vi "ControlSubMM.vi"(0 "ControlPara":dbl[][](array[numeric]), 1 "AxisForceSample":dbl[](array[numeric]), 2 "ChannelSetArray":T1[](array[typedef]) {"Enable" items=["不使能", "使能"]; "Wave" items=["0指令", "正弦波", "方波", "三角波", "常值", "波形数据", "白噪声", "正弦扫频", "梯度加载", "VMIC"]; "ChannelType" items=["标准波形跟踪"=1, "扫频测试"=2, "消除多余力"=3, "梯度加载"=4, "载荷谱跟踪"=5, "模拟输入跟踪"=9]; "ChannelStatus" items=["通道关", "位置通道", "加载通道"]}, 3 "syn-error":dbl[](array[numeric]), 5 "Angel":bool[](array[boolean]), 7 "TorqueSample":dbl[](array[numeric]), 9 "Command":dbl[](array[numeric]), 12 "dt":dbl, 13 "Torque":bool[](array[boolean]), 14 "AngleSample":dbl[](array[numeric])) -> (4 "数组":dbl[](array[numeric]))   [LabVIEW 2020]
uses:
  ChannelCommand.ctl
  Control 1.ctl
  WaveType.ctl
  MoterEnable.ctl
  <vilib>/addons/control/pid/pid.llb/PID (DBL Array).vi
  <vilib>/addons/control/pid/NI_PID_pid.lvlib
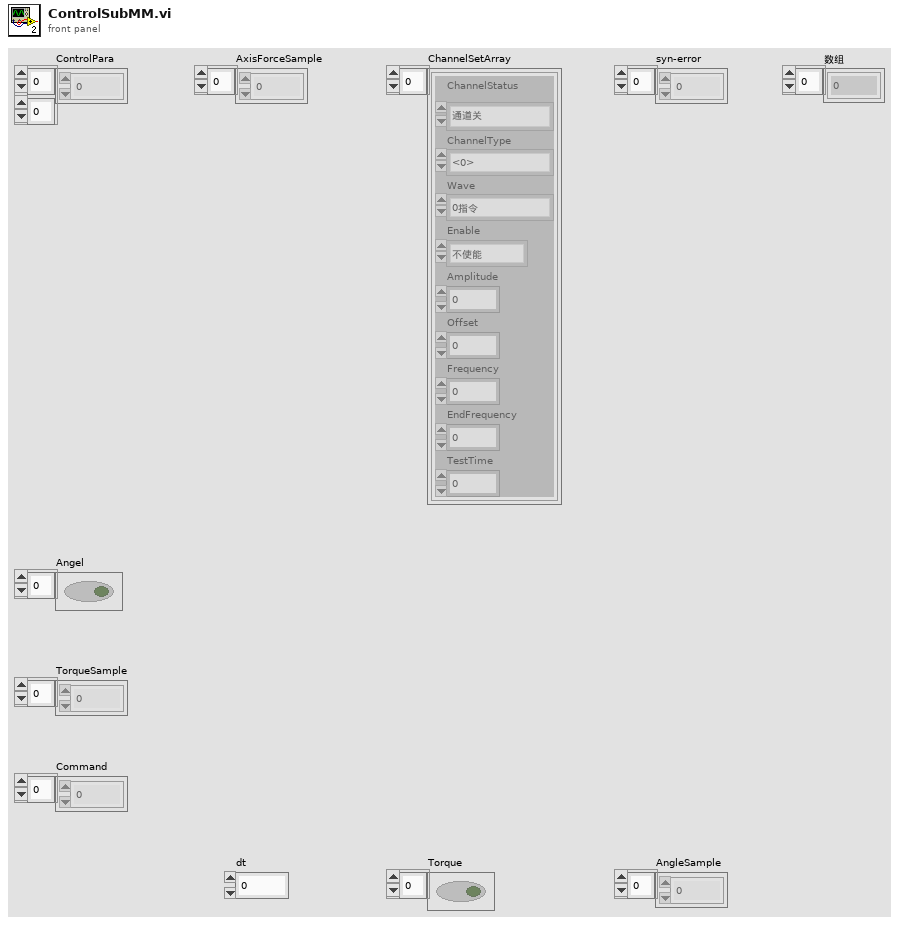
[diagram p1: front panel]
types:
  T1 = typedef "ChannelCommand.ctl" = cluster{"ChannelStatus":T2, "ChannelType":i32, "Wave":T3, "Enable":T4, "Amplitude":dbl, "Offset":dbl, "Frequency":dbl, "EndFrequency":dbl, "TestTime":dbl}
  T2 = typedef "Control 1.ctl" = i32
  T3 = typedef "WaveType.ctl" = i32
  T4 = typedef "MoterEnable.ctl" = u16
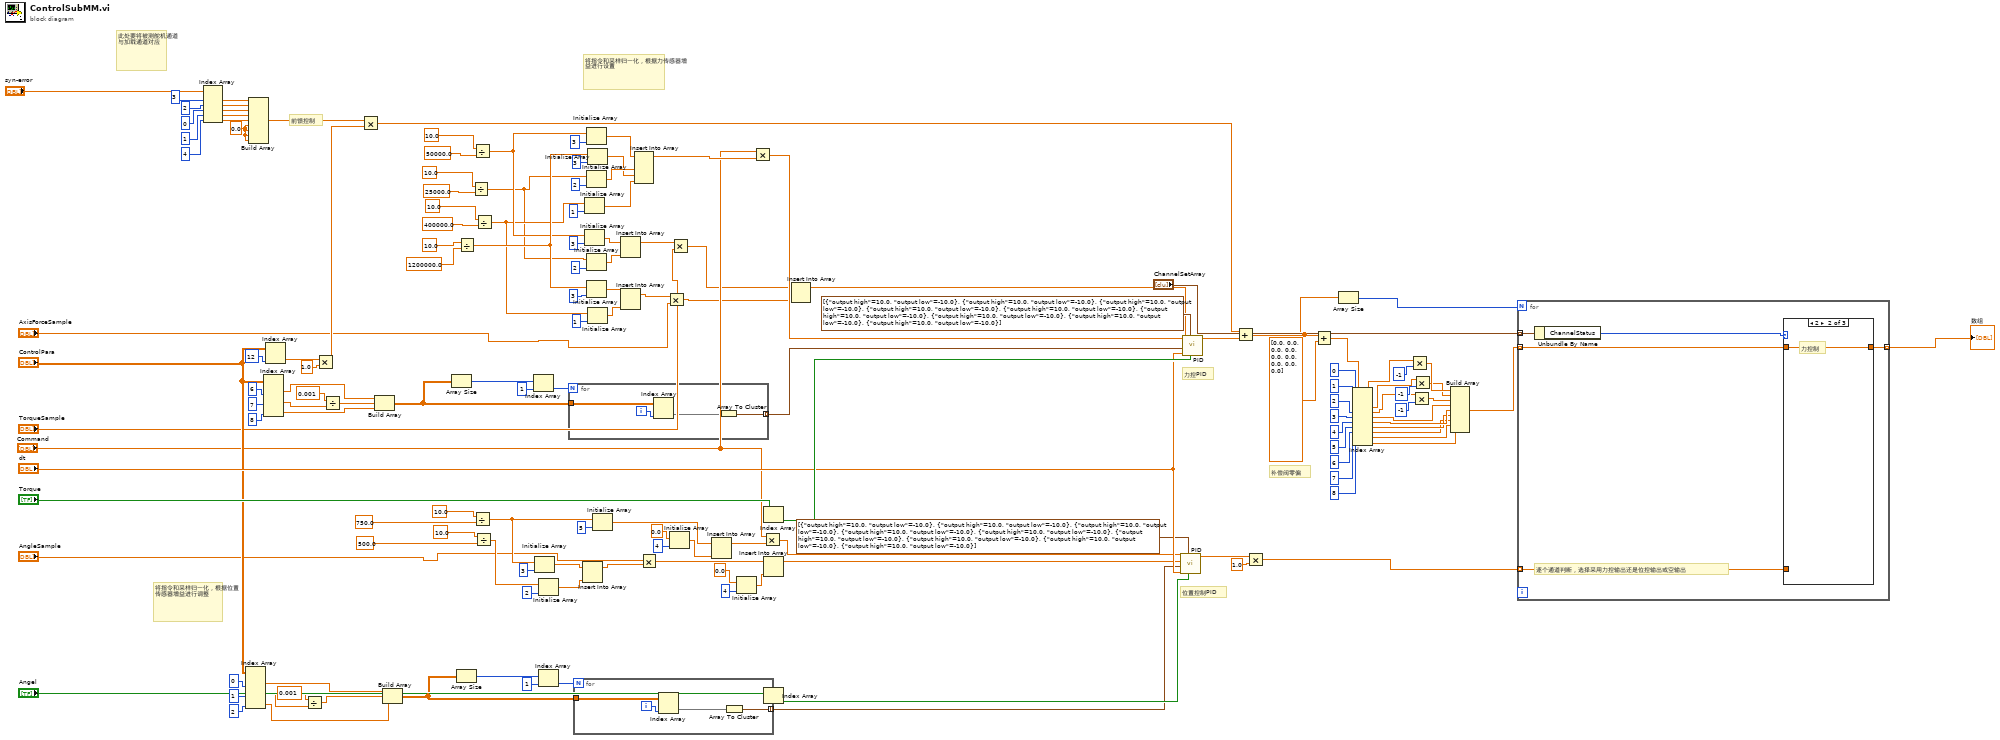
[diagram p0: block diagram]
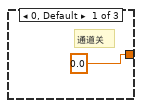
[diagram p2: hidden frame]
diagram:
  w94 = 0.0
  # "补偿阀零偏"
  # "此处要将被测舵机通道与加载通道对应"
  # "将指令和采样归一化，根据力传感器增益进行设置"
  # "将指令和采样归一化，根据位置传感器增益进行调整"
  # "位置控制PID"
  # "力控PID"
  # "前馈控制"
  n1 = Index Array(array="syn-error", index #1=3 ("索引"), index #2=2 ("索引"), index #3=0 ("索引"), index #4=1 ("索引"), index #5=4 ("索引")) -> (element #1=w89:dbl, element #2=w90:dbl, element #3=w91:dbl, element #4=w92:dbl, element #5=w93:dbl)
  n2 = Index Array(array="ControlPara", index (col) #1=0 ("禁用的索引 (列)"), index (col) #2=1 ("索引 (列)"), index (col) #3=2 ("索引 (列)")) -> (element #1=w108:dbl[], element #2=w123:dbl[], element #3=w109:dbl[])  [unwired: 3 in]
  n3 = Build Array(w89, w90, w91, w92, w93, w94, w94, w94, w94) -> (w97:dbl[])
  n4 = Index Array(array="ControlPara", index (col) #1=6 ("禁用的索引 (列)"), index (col) #2=7 ("索引 (列)"), index (col) #3=8 ("索引 (列)")) -> (element #1=w73:dbl[], element #2=w120:dbl[], element #3=w74:dbl[])  [unwired: 3 in]
  n5 = Index Array(array="ControlPara", index (col)=12 ("禁用的索引 (列)")) -> (element=w82:dbl[])  [unwired: 1 in]
  n6 = Divide(x=0.001, y=w123) -> (x/y=w124:dbl[])
  n7 = Multiply(x=w82, y=1.0) -> (x*y=w96:dbl[])
  n8 = Divide(x=0.001, y=w120) -> (x/y=w121:dbl[])
  n9 = Multiply(x=w97, y=w96) -> (x*y=w140:dbl[])
  n10 = Build Array(w73, w121, w74) -> (w78:dbl[][])
  n11 = Build Array(w108, w124, w109) -> (w113:dbl[][])
  n12 = Array Size(array=w78) -> (size(s)=w75:i32[])
  n13 = Array Size(array=w113) -> (size(s)=w110:i32[])
  n14 = Divide(x=10.0 ("元素"), y=1200000.0) -> (x/y=w144:dbl)
  n15 = Divide(x=10.0 ("元素"), y=25000.0) -> (x/y=w44:dbl)
  n16 = Divide(x=10.0 ("元素"), y=50000.0) -> (x/y=w125:dbl)
  n17 = Divide(x=10.0 ("元素"), y=750.0) -> (x/y=w149:dbl)
  n18 = Divide(x=10.0 ("元素"), y=500.0) -> (x/y=w58:dbl)
  n19 = Divide(x=10.0 ("元素"), y=400000.0) -> (x/y=w45:dbl)
  n20 = Index Array(array=w75, index=1 ("索引")) -> (element=w77:i32)
  n21 = Initialize Array(w149, 3 ("维数大小")) -> (w57:dbl[])
  n22 = Initialize Array(w58, 2 ("维数大小")) -> (w56:dbl[])
  n23 = Index Array(array=w110, index=1 ("索引")) -> (element=w112:i32)
  n24 = for {
    N: w77 -> [_]
    tunnel: w78 -> [w153]
    tunnel: [w150] -> w79 mode=indexing
    i -> [w151]
    n25 = Index Array(array=w153, index (col)=w151) -> (element=w152:dbl[])  [unwired: 1 in]
    n26 = Array To Cluster(array=w152) -> (cluster=w150:cluster{"[0]":dbl, "[1]":dbl, "[2]":dbl})
  }
  n27 = for {
    N: w112 -> [_]
    tunnel: w113 -> [w157]
    tunnel: [w154] -> w114 mode=indexing
    i -> [w155]
    n28 = Index Array(array=w157, index (col)=w155) -> (element=w156:dbl[])  [unwired: 1 in]
    n29 = Array To Cluster(array=w156) -> (cluster=w154:cluster{"[0]":dbl, "[1]":dbl, "[2]":dbl})
  }
  n30 = Insert Into Array(array=w57, new element=w56) -> (w55:dbl[])  [unwired: 1 in]
  n31 = Initialize Array(w45, 1 ("维数大小")) -> (w41:dbl[])
  n32 = Initialize Array(w125, 3 ("维数大小")) -> (w38:dbl[])
  n33 = Initialize Array(w125, 3 ("维数大小")) -> (w42:dbl[])
  n34 = Initialize Array(w144, 3 ("维数大小")) -> (w36:dbl[])
  n35 = Initialize Array(w44, 2 ("维数大小")) -> (w40:dbl[])
  n36 = Initialize Array(w44, 2 ("维数大小")) -> (w37:dbl[])
  n37 = Initialize Array(w144, 3 ("维数大小")) -> (w39:dbl[])
  n38 = Initialize Array(w45, 1 ("维数大小")) -> (w35:dbl[])
  n39 = Initialize Array(w149, 5 ("维数大小")) -> (w100:dbl[])
  n40 = Insert Into Array(array=w38, new element=w37) -> (w33:dbl[])  [unwired: 1 in]
  n41 = Insert Into Array(array=w36, new element=w35) -> (w30:dbl[])  [unwired: 1 in]
  n42 = Insert Into Array(array=w42, new element #1=w40, new element #2=w39, new element #3=w41) -> (w63:dbl[])  [unwired: 1 in]
  n43 = Multiply(x="AngleSample", y=w55) -> (x*y=w132:dbl[])
  n44 = Multiply(x=w30, y="AxisForceSample") -> (x*y=w28:dbl[])
  n45 = Initialize Array(0.0 ("元素"), 4 ("维数大小")) -> (w127:dbl[])
  n46 = Multiply(x=w33, y="TorqueSample") -> (x*y=w31:dbl[])
  n47 = Insert Into Array(array=w100, new element=w127) -> (w101:dbl[])  [unwired: 1 in]
  n48 = Initialize Array(0.0 ("元素"), 4 ("维数大小")) -> (w133:dbl[])
  n49 = Multiply(x="Command", y=w63) -> (x*y=w66:dbl[])
  n50 = Multiply(x="Command", y=w101) -> (x*y=w104:dbl[])
  n51 = Index Array(array="Torque") -> (element=w146:bool)  [unwired: 1 in]
  n52 = Insert Into Array(array=w132, new element=w133) -> (w134:dbl[])  [unwired: 1 in]
  n53 = Index Array(array="Angel") -> (element=w148:bool)  [unwired: 1 in]
  n54 = Insert Into Array(array=w31, new element=w28) -> (w69:dbl[])  [unwired: 1 in]
  n55 = call-poly <vilib>:"PID.vi"("reinitialize? (F)"=w148, "output range"=cluster{"output high":dbl, "output low":dbl}[] [{"output high"=10.0, "output low"=-10.0}, {"output high"=10.0, "output low"=-10.0}, {"output high"=10.0, "output low"=-10.0}, {"output high"=10.0, "output low"=-10.0}, {"output high"=10.0, "output low"=-10.0}, {"output high"=10.0, "output low"=-10.0}, {"output high"=10.0, "output low"=-10.0}, {"output high"=10.0, "output low"=-10.0}, {"output high"=10.0, "output low"=-10.0}], "dt (s)"="dt", "PID gains"=w114, "process variable"=w134, "setpoint"=w104) -> ("output"=w135:dbl[])  [unwired: 4 in, 1 out]
  n56 = call-poly <vilib>:"PID.vi"("reinitialize? (F)"=w146, "output range"=cluster{"output high":dbl, "output low":dbl}[] [{"output high"=10.0, "output low"=-10.0}, {"output high"=10.0, "output low"=-10.0}, {"output high"=10.0, "output low"=-10.0}, {"output high"=10.0, "output low"=-10.0}, {"output high"=10.0, "output low"=-10.0}, {"output high"=10.0, "output low"=-10.0}, {"output high"=10.0, "output low"=-10.0}, {"output high"=10.0, "output low"=-10.0}, {"output high"=10.0, "output low"=-10.0}], "dt (s)"="dt", "PID gains"=w79, "process variable"=w69, "setpoint"=w66) -> ("output"=w98:dbl[])  [unwired: 4 in, 1 out]
  n57 = Add(x=w140, y=w98) -> (x+y=w43:dbl[])
  n58 = Multiply(x=w135, y=1.0) -> (x*y=w139:dbl[])
  n59 = Add(x=w43, y=dbl[] [0.0, 0.0, 0.0, 0.0, 0.0, 0.0, 0.0, 0.0, 0.0]) -> (x+y=w11:dbl[])
  n60 = Array Size(array=w43) -> (size(s)=w138:i32)
  n61 = Index Array(array=w11, index #1=0 ("索引"), index #2=1 ("索引"), index #3=2 ("索引"), index #4=3 ("索引"), index #5=4 ("索引"), index #6=5 ("索引"), index #7=6 ("索引"), index #8=7 ("索引"), index #9=8 ("索引")) -> (element #1=w10:dbl, element #2=w9:dbl, element #3=w8:dbl, element #4=w7:dbl, element #5=w6:dbl, element #6=w5:dbl, element #7=w4:dbl, element #8=w3:dbl, element #9=w2:dbl)
  n62 = Multiply(x=w10, y=-1) -> (x*y=w25:dbl)
  n63 = Multiply(x=w8, y=-1) -> (x*y=w21:dbl)
  n64 = Multiply(x=w9, y=-1) -> (x*y=w23:dbl)
  n65 = Build Array(w25, w23, w21, w7, w6, w5, w4, w3, w2) -> (w1:dbl[])
  n66 = for {
    N: w138 -> [_]
    tunnel: w1 -> [w160] mode=indexing
    tunnel: w139 -> [w158] mode=indexing
    tunnel: "ChannelSetArray" -> [w162] mode=indexing
    tunnel: [w159] -> w142 mode=indexing
    # "逐个通道判断，选择采用力控输出还是位控输出或空输出"
    n67 = Unbundle By Name(w162) -> ("ChannelStatus"=w161:T2)
    n68 = case shown="2" w161 {
      tunnel: w158 -> [_ _ w165]
      tunnel: w160 -> [_ w164 _]
      tunnel: [0.0 w164 w165] -> w159
      frame 0, Default {
        # "通道关"
      }
      frame 2 {
        # "力控制"
      }
      frame 1 {
        # "位置控制"
      }
    }
  }
  "数组" <- w142
